vi "Get visa 1d DBL data.vi"(7 "VISA resource name":refnum<visa-resource-name>, 8 "error in (no error)":errorcluster, 9 "Name":string, 10 "Mag Lab Parameters in":refnum<class "Mag Lab Parameters.lvclass">, 11 "HPNeworkAnalyzer in":refnum<class "HPNeworkAnalyzer.lvclass">) -> (0 "error out":errorcluster, 1 "Channel data":dbl[](array[numeric]), 2 "Channel names":string[](array[string]), 3 "HPNeworkAnalyzer out":refnum<class "HPNeworkAnalyzer.lvclass">, 5 "VISA resource name out":refnum<visa-resource-name>)   [LabVIEW 2015, in "HPNeworkAnalyzer.lvclass"]
uses:
  HPNeworkAnalyzer.lvclass
  Mag Lab Properties/Mag Lab Parameters.lvclass
  NHMFL_Core/Libraries/Instruments/GPIB/VISA  Send Receive.vi
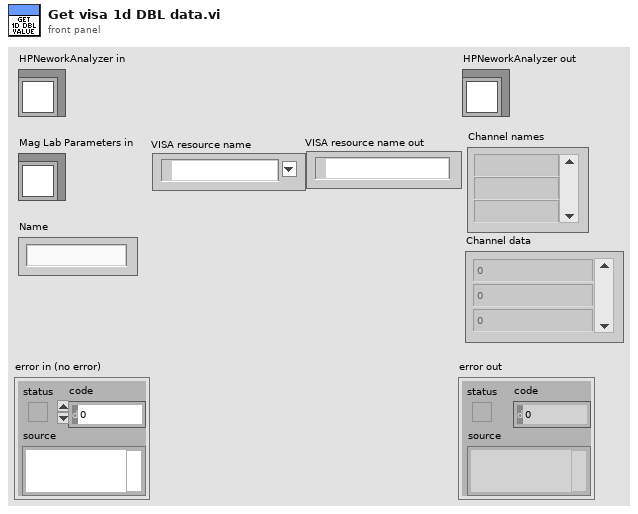
[diagram p1: front panel]
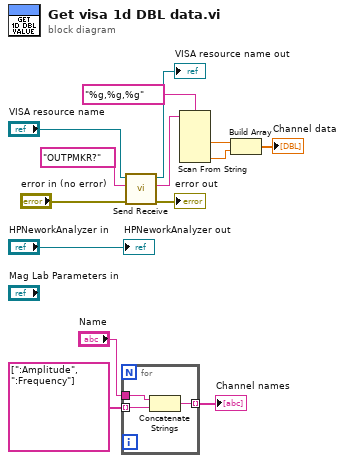
[diagram p0: block diagram]
diagram:
  n1 = for {
    tunnel: "Name" -> [w17]
    tunnel: string[] [":Amplitude", ":Frequency"] -> [w16] mode=indexing
    tunnel: [w15] -> w12 mode=indexing
    n2 = Concatenate Strings(w17, w16) -> (w15:string)
  }
  "Channel names" <- w12
  n3 = call-poly "Send Receive.vi"("error in (no error)"="error in (no error)", "data string in"="OUTPMKR?" ("data"), "VISA Resource Name"="VISA resource name") -> ("error out"=→"error out":errorcluster, "data string out"=w9:string, "VISA Resource Name Out"=→"VISA resource name out":refnum<visa-resource-name>)  [unwired: 6 in]
  n4 = Scan From String(format string="%g,%g,%g", input string=w9) -> (output 1=w7:dbl, output 3=w6:dbl)  [unwired: 6 in, 3 out]
  n5 = Build Array(w7, w6) -> (→"Channel data":dbl[])
  "HPNeworkAnalyzer out" <- "HPNeworkAnalyzer in"
